vi "Custom-preview-graph-override.vi"(5 "Unit display D 2":refnum<vi>, 7 "enabled?":bool, 8 "Data":dbl[](array[numeric]), 9 "Labels":string[](array[string]), 11 "last tick":u32) -> (0 "Data out":dbl[](array[numeric]), 1 "Labels out":string[](array[string]), 3 "new tick":u32)   [LabVIEW 2013]
panel:
  out "Chart history size":i32
  out "last value Wh":dbl
  in  "ignore all over x ms":u32=10000
  out "td":u32
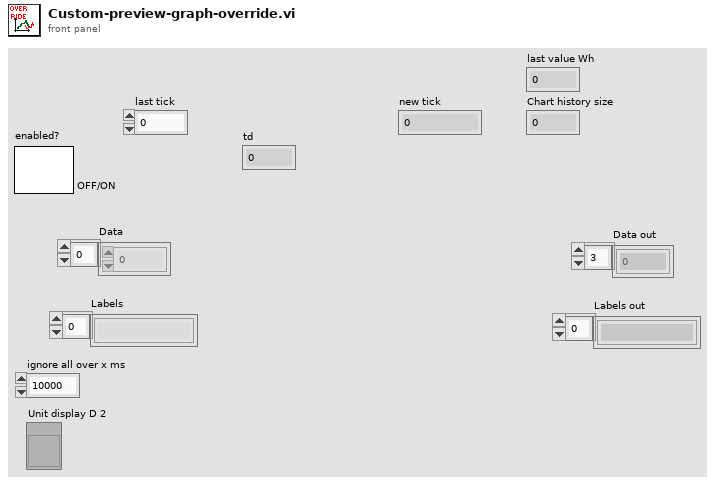
[diagram p1: front panel]
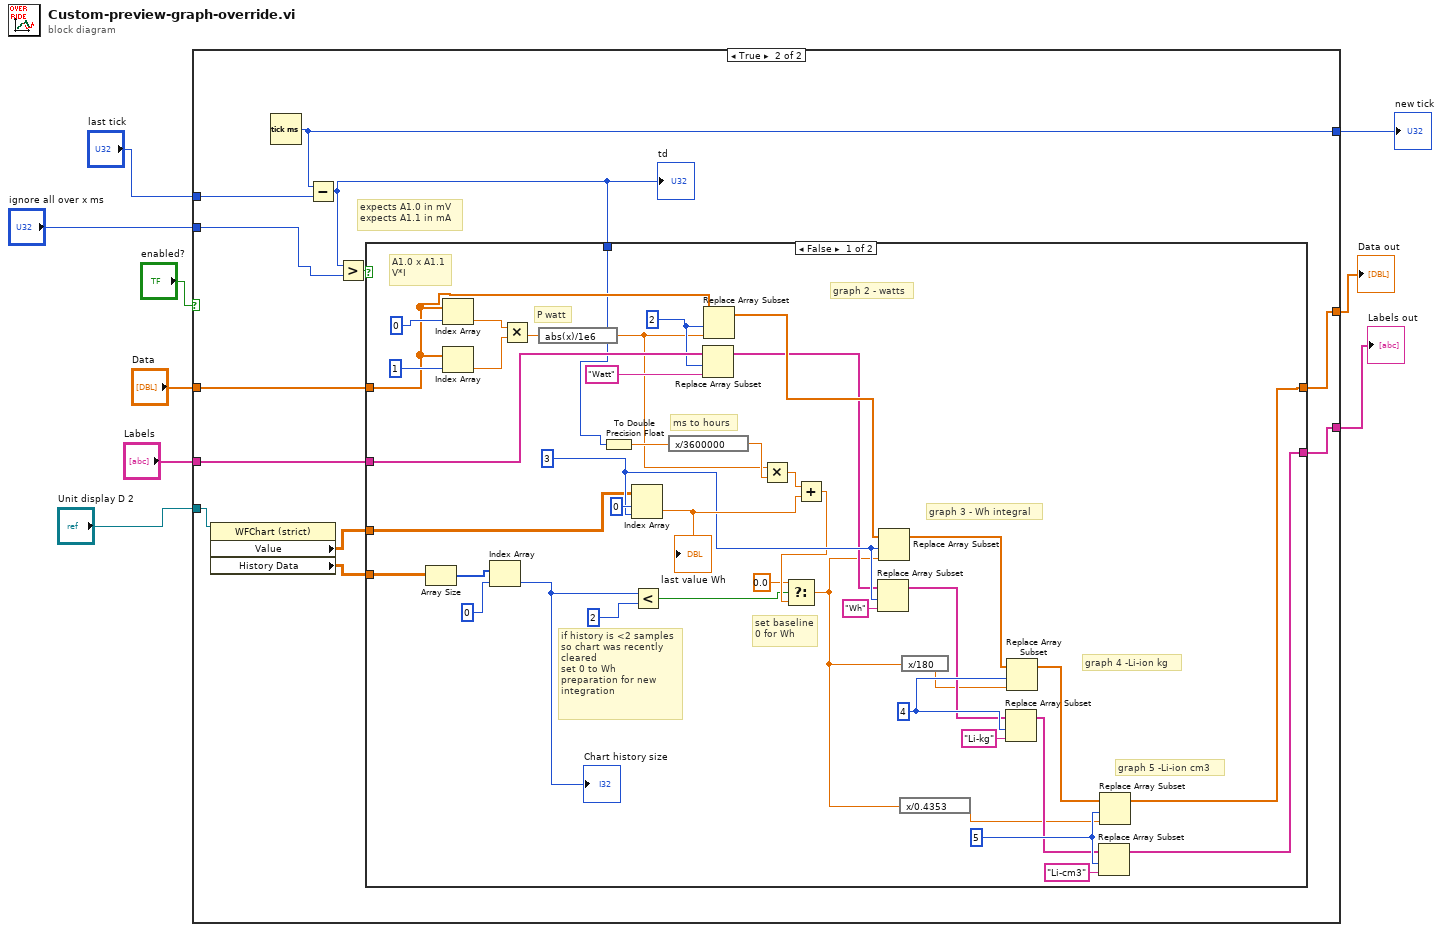
[diagram p0: block diagram]
diagram:
  n1 = case shown="True" "enabled?" {
    tunnel: [_ w23] -> w9
    tunnel: [w11 w19] -> w7
    tunnel: "Data" -> [w11 w18]
    tunnel: [w10 w17] -> w5
    tunnel: "Labels" -> [w10 w16]
    tunnel: "last tick" -> [_ w22]
    tunnel: "ignore all over x ms" -> [_ w20]
    tunnel: "Unit display D 2" -> [_ w14]
    frame False {
    }
    frame True {
      # "expects A1.0 in mV\nexpects A1.1 in mA"
      n2 = property class="WFChart (strict)"(reference=w14) -> ("Value"=w13:dbl[][], "History Data"=w12:dbl[][])  [unwired: 1 in, 2 out]
      n3 = Tick Count (ms)() -> (millisecond timer value=w23:u32)
      n4 = Subtract(x=w23, y=w22) -> (x-y=w15:u32)
      "td" <- w15
      n5 = Greater?(x=w15, y=w20) -> (0:w21:bool)
      n6 = case shown="False" w21 {
        tunnel: [w38 w67] -> w19
        tunnel: w18 -> [w61 w67]
        tunnel: [w37 w66] -> w17
        tunnel: w16 -> [w60 w66]
        tunnel: w15 -> [w55 _]
        tunnel: w13 -> [w33 _]
        tunnel: w12 -> [w29 _]
        frame False {
          w43 = 5 ("disabled index (col)")
          w44 = 4 ("disabled index (col)")
          w49 = 3 ("disabled index (col)")
          w57 = 2 ("index")
          # "if history is <2 samples\nso chart was recently\ncleared\nset 0 to Wh\npreparation for new\nintegration"
          # "set baseline\n0 for Wh"
          # "graph 5 -Li-ion cm3"
          # "graph 4 -Li-ion kg"
          # "ms to hours"
          # "graph 3 - Wh integral"
          # "graph 2 - watts"
          # "P watt"
          # "A1.0 x A1.1\nV*I"
          n7 = Array Size(array=w29) -> (size(s)=w28:i32[])
          n8 = Index Array(array=w61, index=0) -> (element=w63:dbl)
          n9 = Index Array(array=w61, index=1) -> (element=w62:dbl)
          n10 = Index Array(array=w28, index=0) -> (element=w26:i32)
          "Chart history size" <- w26
          n11 = Multiply(x=w63, y=w62) -> (x*y=w56:dbl)
          n12 = expression code="abs(x)/1e6"(w56) -> (w34:dbl)
          n13 = To Double Precision Float(number=w55) -> (double precision float=w54:dbl)
          n14 = Index Array(array=w33, index (row)=0, index (col)=w49) -> (element=w51:dbl)
          "last value Wh" <- w51
          n15 = Less?(x=w26, y=2) -> (x < y?=w24:bool)
          n16 = expression code="x/3600000"(w54) -> (w53:dbl)
          n17 = Replace Array Subset(array=w60, new element="Watt" ("new element/subarray"), index=w57) -> (w48:string[])
          n18 = Replace Array Subset(array=w61, new element=w34, index=w57) -> (w50:dbl[])
          n19 = Multiply(x=w34, y=w53) -> (x*y=w52:dbl)
          n20 = Add(x=w52, y=w51) -> (x+y=w31:dbl)
          n21 = Select(t=0.0, s=w24, f=w31) -> (s? t:f=w32:dbl)
          n22 = Replace Array Subset(array=w48, new element="Wh" ("new element/subarray"), index=w49) -> (w40:string[])
          n23 = Replace Array Subset(array=w50, new element=w32, index=w49) -> (w42:dbl[])
          n24 = expression code="x/0.4353"(w32) -> (w35:dbl)
          n25 = expression code="x/180"(w32) -> (w36:dbl)
          n26 = Replace Array Subset(array=w40, new element="Li-kg" ("new element/subarray"), index=w44) -> (w39:string[])
          n27 = Replace Array Subset(array=w42, new element=w36, index=w44) -> (w41:dbl[])
          n28 = Replace Array Subset(array=w39, new element="Li-cm3" ("new element/subarray"), index=w43) -> (w37:string[])
          n29 = Replace Array Subset(array=w41, new element=w35, index=w43) -> (w38:dbl[])
        }
        frame True {
          # "ignore all over 10s"
        }
      }
    }
  }
  "new tick" <- w9
  "Data out" <- w7
  "Labels out" <- w5
